vi "Main_6b refactored.vi"() -> ()   [LabVIEW 2020]
uses:
  0c0f8bb7-c444-485a-b807-04b59ab5f06f.vi
panel:
  out "Position of marker":i32
  in  "Example 5":string="zcfzfwzzqfrljwzlrfnpqdbhtmscgvjw"
  in  "Example 4":string="nznrnfrfntjfmvfwmzdfjlvtqnbhcprsg"
  in  "Example 3":string="mjqjpqmgbljsphdztnvjfqwrcgsmlb"
  in  "Example 2":string="bvwbjplbgvbhsrlpgdmjqwftvncz"
  in  "Puzzle":string="plhlsssjsrscspsffmrffwvfvrvvmbbnjnrnrfnndlnlznlznlnccdbbhvbvgvmvzmzvmzmbbrcclsslzslzzsztzftzzhggnjgnjnhnmnqnqqfdfnnrwnwsnwwvgvqqgpptvtrvvfmmzjzmmjssmwsmmhzzvvwzwcwrcrllpbppdgdvvwqvvsnsrnsncnwntnggwqgqhqrqprqrddjvddqsqhshchfffzddswdsshhcnhnqqfjffvlvwvssdqqwrwvrvhrvrzzgwggcjcgclcwchhzvzmzrrjwjqwwvbwwrmmvmpmzpzgpgsghgrrtmmlfmmnzzmpzzvmvjjsqqshqshsqqgtqggpvvrtttwbbhnbnlbnlnhnthtjhjshhrmrjjlclpprmrnrsrwrbwrwwjnwnbwbhbmbggdbgghllcvlvddzbdbdvdwvdvjvqvcvczvcvclvvrggrngrrwcwbcczgghnhznhnttbcbvcvttrrpbrppndppvvvgvtgvvhfvhhttppjmjllznlnldnldlwlnwlnlttgzzcfcggwmgmqgmmshmhqqdfqfpfqppprzrhrnrhnrrtsrrgpgnpng..."
  in  "Example":string="mjqjpqmgbljsphdztnvjfqwrcgsmlb"
  # "Your device's communication system is correctly detecting packets, but still isn't working. It looks like it also needs to look for messages.\n\nA start-of-message marker is just like a start-of-packet marker, except it consists of 14 distinct characters rather than 4.\n\nHere are the first positions of start-of-message markers for all of the above examples:\n\nmjqjpqmgbljsphdztnvjfqwrcgsmlb: first marker after character 19\nbvwbjplbgvbhsrlpgdmjqwftvncz: first marker after character 23\nnppdvjthqldpwncqszvftbrmjlhg: first marker after character 23\nnznrnfrfntjfmvfwmzdfjlvtqnbhcprsg: first marker after character 29\nzcfzfwzzqfrljwzlrfnpqdbhtmscgvjw: first marker after character 26\nHow many characters need to be processed before the first start-of-message marker is detected?"
  # "3716"
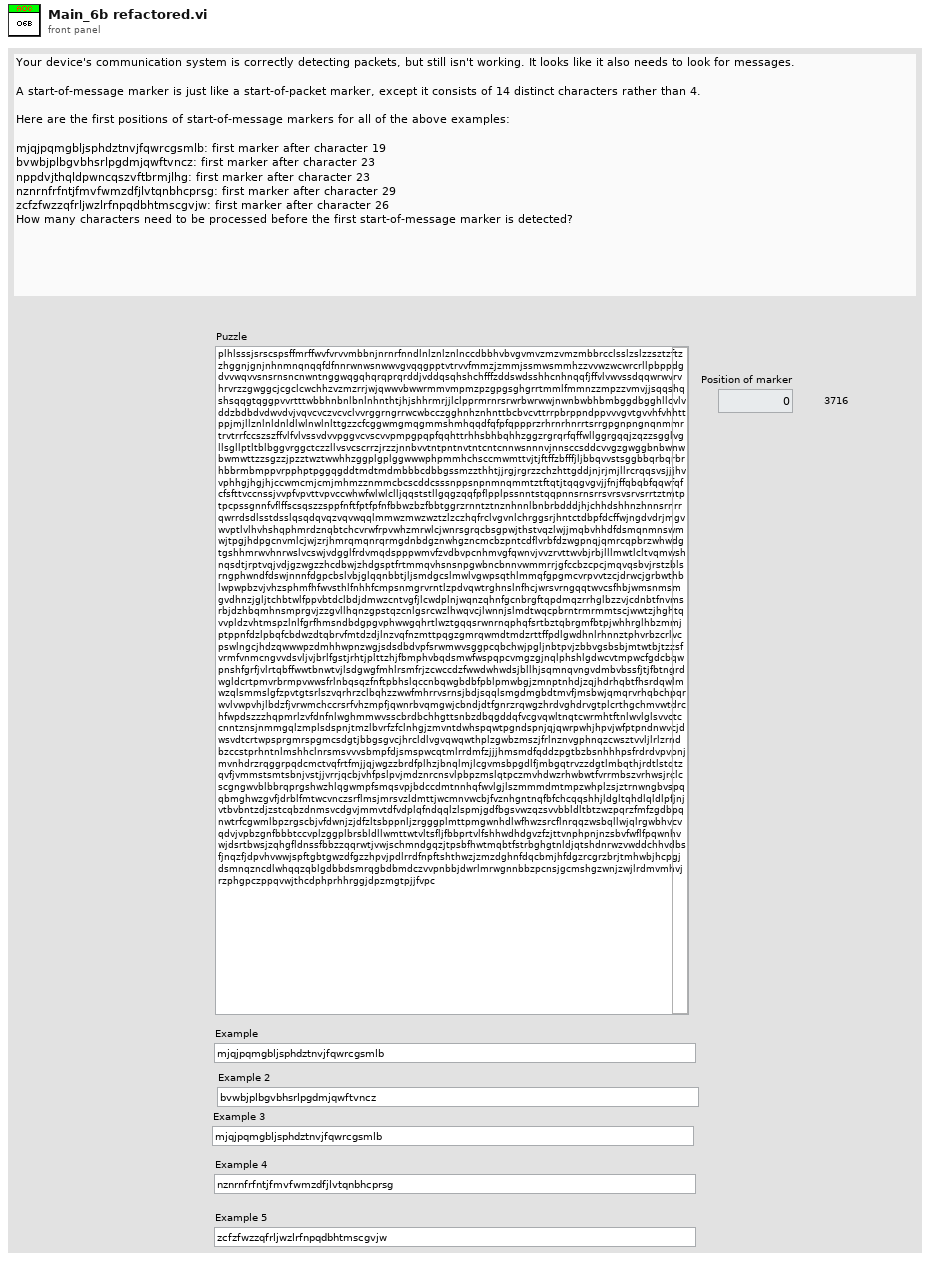
[diagram p1: front panel]
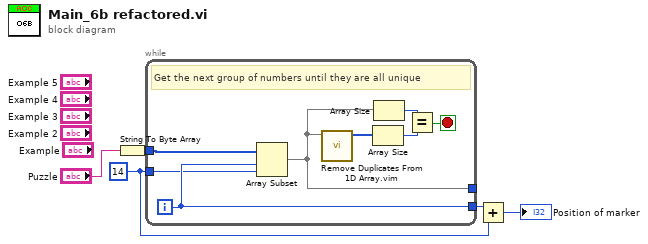
[diagram p0: block diagram]
diagram:
  w1 = 14 ("length")
  n1 = String To Byte Array(string="Puzzle") -> (unsigned byte array=w5:u8[])
  n2 = while {
    tunnel: w5 -> [w13]
    tunnel: [w10] -> _
    tunnel: [w11] -> w4
    tunnel: w1 -> [w7]
    i -> [w11]
    stop <- w6 stop-if-true
    # "Get the next group of numbers until they are all unique"
    n3 = Array Subset(array=w13, index=w11, length=w7) -> (w10:u8[])
    n4 = call "Remove Duplicates From 1D Array.vim"("array"=w10) -> ("array with duplicates removed"=w9:u8[])  [unwired: 10 in]
    n5 = Array Size(array=w9) -> (size(s)=w8:i32)
    n6 = Array Size(array=w10) -> (size(s)=w12:i32)
    n7 = Equal?(x=w12, y=w8) -> (x = y?=w6:bool)
  }
  n8 = Add(x=w4, y=w1) -> (x+y=→"Position of marker":i32)
